vi "FVIR_VESTA_Main.vi"(8 "error in":errorcluster, 10 "VISA resource name":refnum<visa-resource-name>="VESTA_LDO", 11 "Message Queues":T1) -> (0 "error out":errorcluster)   [LabVIEW 2020]
uses:
  Message Queue/All Message Queues.ctl
  Message Queue/Message Cluster.ctl
  Message Queue/Enqueue Message (Single).vi
  Message Queue/Message Queue.lvlib
panel:
  out "Loop Count":i32
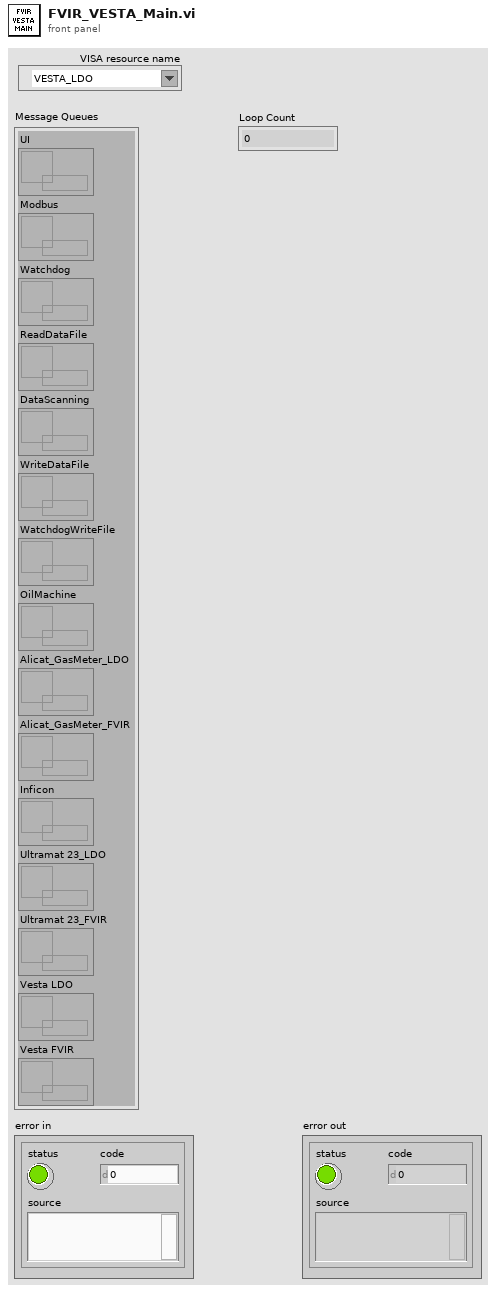
[diagram p1: front panel]
types:
  T1 = typedef "Message Queue.lvlib/All Message Queues.ctl" = cluster{"UI":refnum<queue>, "Modbus":refnum<queue>, "Watchdog":refnum<queue>, "ReadDataFile":refnum<queue>, "DataScanning":refnum<queue>, "WriteDataFile":refnum<queue>, "WatchdogWriteFile":refnum<queue>, "OilMachine":refnum<queue>, "Alicat_GasMeter_LDO":refnum<queue>, "Inficon":refnum<queue>, "Ultramat 23_LDO":refnum<queue>, "Alicat_GasMeter_FVIR":refnum<queue>, "Ultramat 23_FVIR":refnum<queue>, "Vesta LDO":refnum<queue>, "Vesta FVIR":refnum<queue>}
  T2 = typedef "Vesta Info.ctl" = cluster{"Temp_W_Raw_U":u16, "Temp_W_Raw_L":u16, "Temperature Water (F)":dbl, "Temperature Water Compensated (F)":dbl, "Temperature Ambient (F)":dbl, "Setpoint Location (F)":dbl, "Heat Request":string, "Fault Ram":string, "PWM DCDC Value":u16, "Pilot Voltage (mV)":dbl, "Setpoint Actual (F)":dbl, "Differential Actual (F)":dbl, "Setpoint User (F)":dbl, "Differential User (F)":dbl, "Termperature FIltered -TCO (F)":dbl, "Temp_C_Raw_1 - Sensor Voltage":string, "Temp_C_Raw_2 - Sensor Voltage":string, "Chamber Sensor Temperature (F)":dbl, "LDO Base Temperature (F)":dbl, "LDO Timer (sec)":i16, "Disabled (0)":bool, "Warming (1)":bool, "Heating (2)":bool, "Cooling Data Write (3)":bool, "Cooling (4)":bool, "Data Read (5)":bool, "N/A":bool, "Temperature Trip (7)":bool}
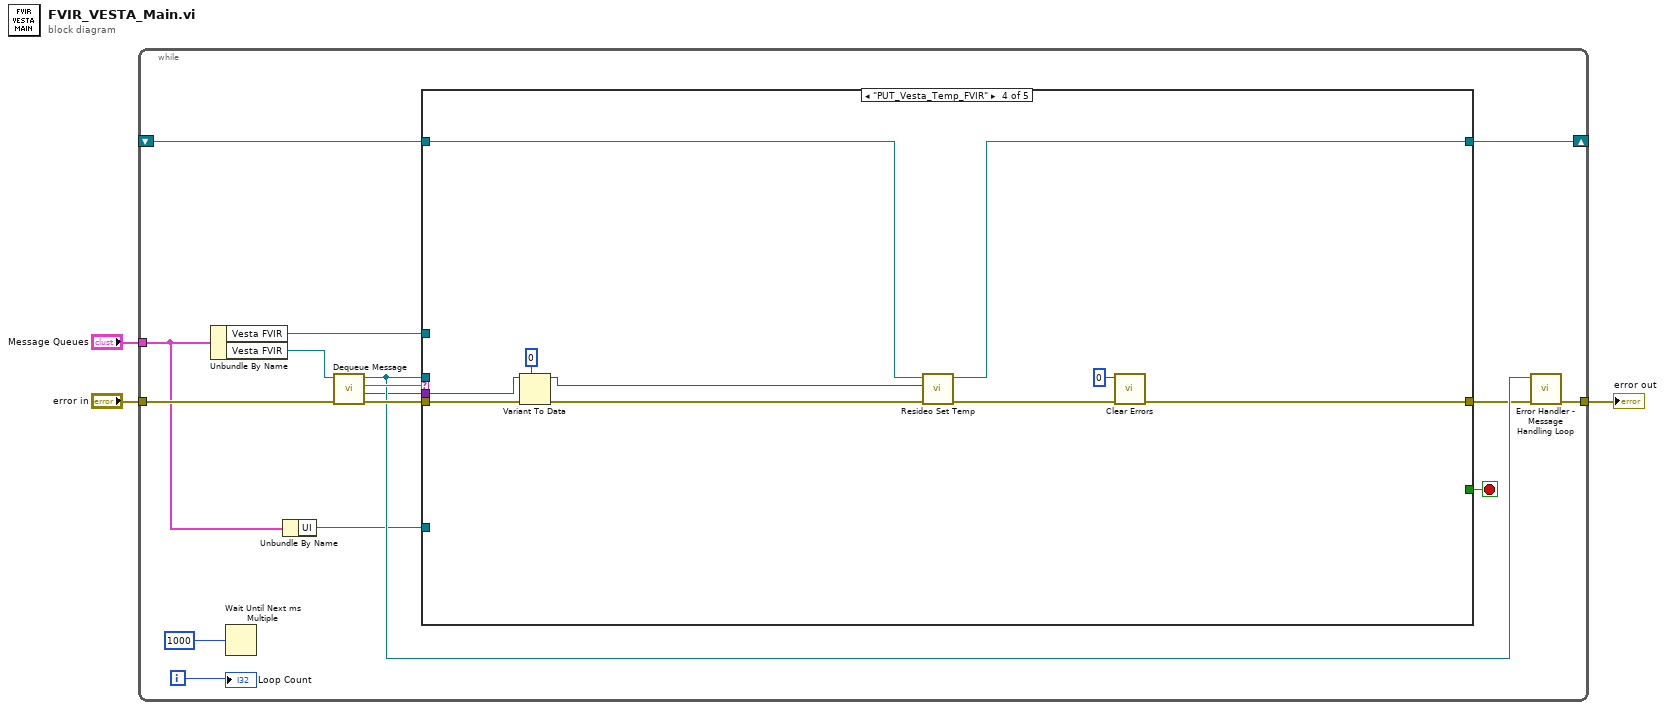
[diagram p0: block diagram]
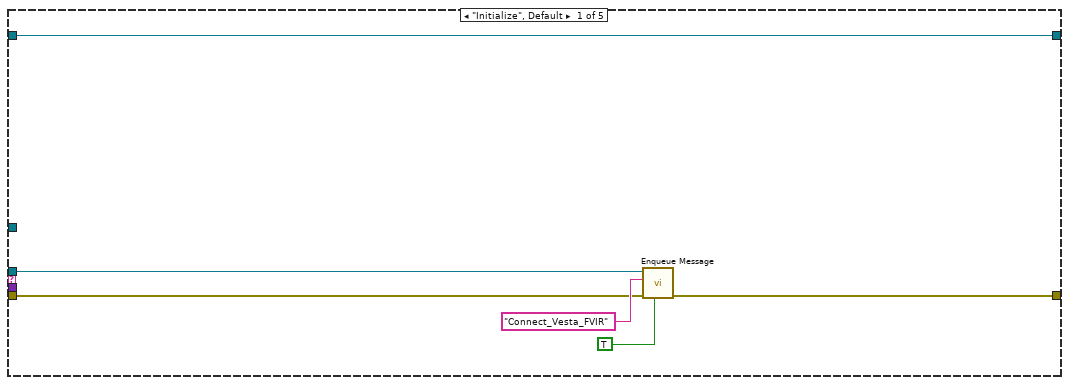
[diagram p2: hidden frame]
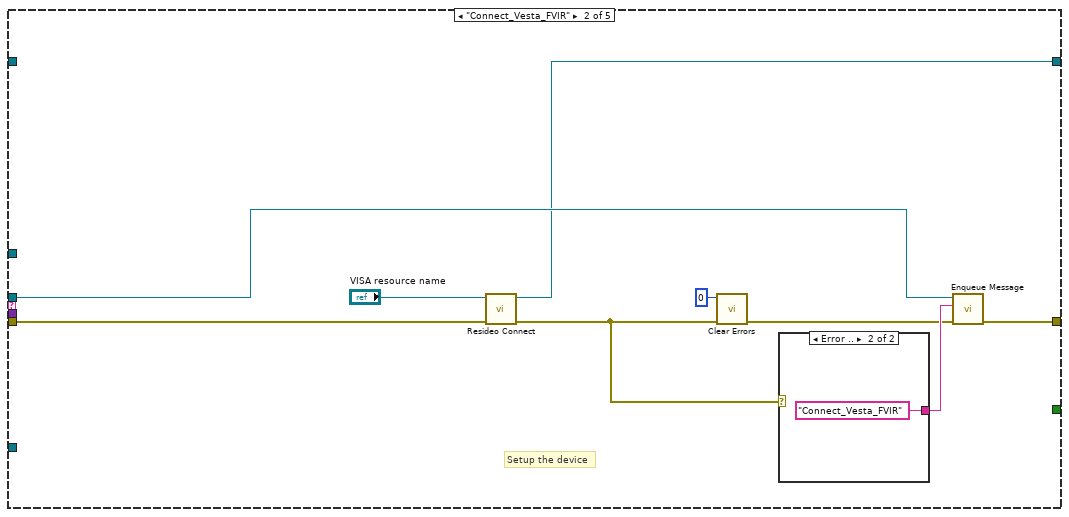
[diagram p3: hidden frame]
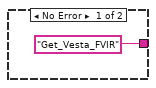
[diagram p4: hidden frame]
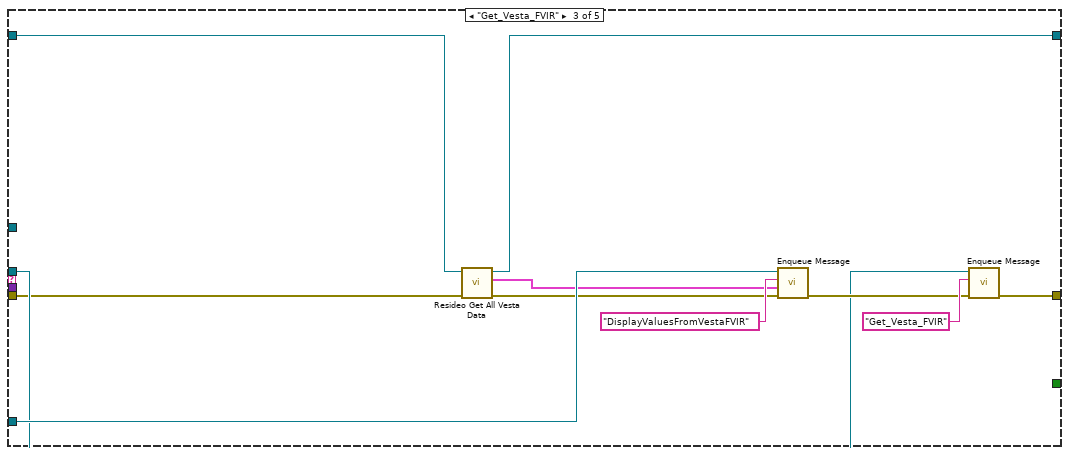
[diagram p5: hidden frame]
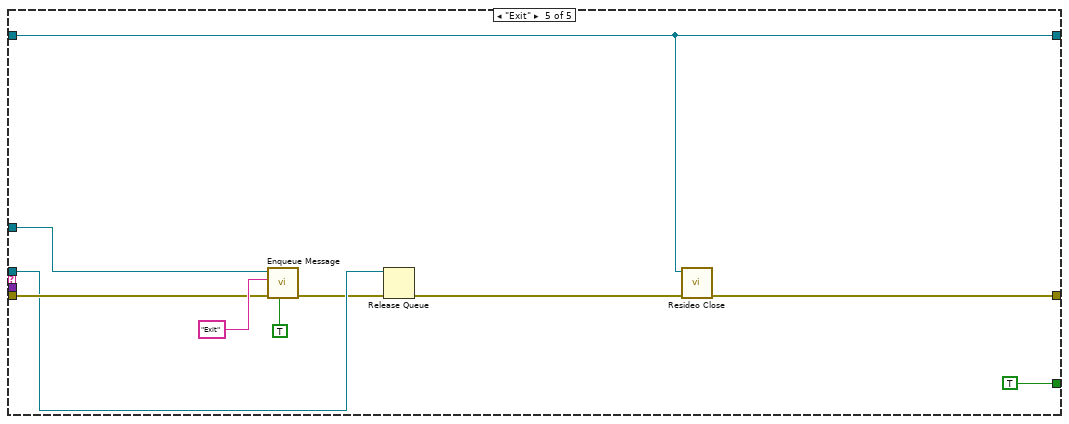
[diagram p6: hidden frame]
diagram:
  n1 = while {
    tunnel: "Message Queues" -> [w9]
    tunnel: "error in" -> [w18]
    tunnel: [w12] -> w1
    shift-right: [w7] -> _
    shift-left: _ -> [w6]
    i -> [w5]
    stop <- w15 stop-if-true
    n2 = Unbundle By Name(w9) -> ("Vesta FVIR"=w14:refnum<queue>, "Vesta FVIR"=w19:refnum<queue>)
    n3 = Wait Until Next ms Multiple(millisecond multiple=u32 1000) -> ()  [unwired: 1 out]
    n4 = Unbundle By Name(w9) -> ("UI"=w8:refnum<queue>)
    n5 = call "Dequeue Message.vi"("error in (no error)"=w18, "Message Queue"=w19) -> ("error out"=w16:errorcluster, "Message Data"=w4:variant, "Message"=w17:string, "dup Message Queue"=w13:refnum<queue>)  [unwired: 6 in]
    n6 = case shown="\"PUT_Vesta_Temp_FVIR\"" w17 {
      tunnel: w16 -> [w24 w29 w41 w54 w63]
      tunnel: [w23 w33 w43 w49 w59] -> w11
      tunnel: [_ _ _ _ TRUE] -> w15
      tunnel: w14 -> [_ _ _ _ w64]
      tunnel: w13 -> [w22 w32 w42 _ w62]
      tunnel: w8 -> [_ _ w46 _ _]
      tunnel: [w21 w30 w39 w56 w58] -> w7
      tunnel: w6 -> [w21 _ w40 w57 w58]
      tunnel: w4 -> [_ _ _ w52 _]
      frame "Initialize", Default {
        n7 = call-poly "Enqueue Message.vi"("Priority Message? (F)"=TRUE, "error in (no error)"=w24, "Message"="Connect_Vesta_FVIR", "Message Queue"=w22) -> ("error out"=w23:errorcluster)  [unwired: 6 in, 1 out]
      }
      frame "Connect_Vesta_FVIR" {
        # "Setup the device"
        n8 = call "Resideo Connect.vi"("error in (no error)"=w29, "VISA Refnum in"="VISA resource name") -> ("error out"=w26:errorcluster, "Modbus Master out"=w30:refnum<class "Modbus Master.lvclass">)  [unwired: 8 in]
        n9 = call <vilib>:"Clear Errors.vi"("error in (no error)"=w26, "specific error code to clear (0: all)"=0) -> ("error out"=w28:errorcluster)  [unwired: 4 in, 1 out]
        n10 = case shown="Error .." w26 {
          tunnel: ["Get_Vesta_FVIR" ("Message") "Connect_Vesta_FVIR" ("Message")] -> w34
          frame No Error {
          }
          frame Error {
          }
        }
        n11 = call-poly "Enqueue Message.vi"("error in (no error)"=w28, "Message"=w34, "Message Queue"=w32) -> ("error out"=w33:errorcluster)  [unwired: 7 in, 1 out]
      }
      frame "Get_Vesta_FVIR" {
        n12 = call "Resideo Get All Vesta Data.vi"("error in (no error)"=w41, "Modbus Master in"=w40) -> ("error out"=w38:errorcluster, "Vesta Data Output"=w37:T2, "Modbus Master out"=w39:refnum<class "Modbus Master.lvclass">)  [unwired: 7 in]
        n13 = call-poly "Enqueue Message.vi"("error in (no error)"=w38, "Message Data"=w37, "Message"="DisplayValuesFromVestaFVIR", "Message Queue"=w46) -> ("error out"=w44:errorcluster)  [unwired: 6 in, 1 out]
        n14 = call-poly "Enqueue Message.vi"("error in (no error)"=w44, "Message"="Get_Vesta_FVIR", "Message Queue"=w42) -> ("error out"=w43:errorcluster)  [unwired: 7 in, 1 out]
      }
      frame "PUT_Vesta_Temp_FVIR" {
        n15 = Variant To Data(error in=w54, type=u16 0, Variant=w52) -> (data=w51:u16, error out=w53:errorcluster)
        n16 = call "Resideo Set Temp.vi"("error in (no error)"=w53, "Temperature Setpoint"=w51, "Modbus Master in"=w57) -> ("error out"=w50:errorcluster, "Modbus Master out"=w56:refnum<class "Modbus Master.lvclass">)  [unwired: 7 in]
        n17 = call <vilib>:"Clear Errors.vi"("error in (no error)"=w50, "specific error code to clear (0: all)"=0) -> ("error out"=w49:errorcluster)  [unwired: 4 in, 1 out]
      }
      frame "Exit" {
        n18 = call-poly "Enqueue Message.vi"("Priority Message? (F)"=TRUE, "error in (no error)"=w63, "Message"="Exit", "Message Queue"=w64) -> ("error out"=w61:errorcluster)  [unwired: 6 in, 1 out]
        n19 = Release Queue(queue=w62, error in (no error)=w61) -> (error out=w60:errorcluster)  [unwired: 1 in, 2 out]
        n20 = call "Resideo Close.vi"("error in (no error)"=w60, "Modbus Master in"=w58) -> ("error out"=w59:errorcluster)  [unwired: 9 in]
      }
    }
    n21 = call "Error Handler - Message Handling Loop.vi"("error in (no error)"=w11, "Message Queue"=w13) -> ("dup error in"=w12:errorcluster)  [unwired: 8 in, 1 out]
    "Loop Count" <- w5
  }
  "error out" <- w1
